vi "getType.vi"(8 "error in (no error)":errorcluster, 11 "Wire in":refnum<class "TextDecoration.lvclass">) -> (0 "error out":errorcluster, 2 "type":string, 3 "Wire out":refnum<class "TextDecoration.lvclass">)   [LabVIEW 2023, in "TLC_Scripto.lvlib" / "TextDecoration.lvclass"]
uses:
  TextDecoration.lvclass
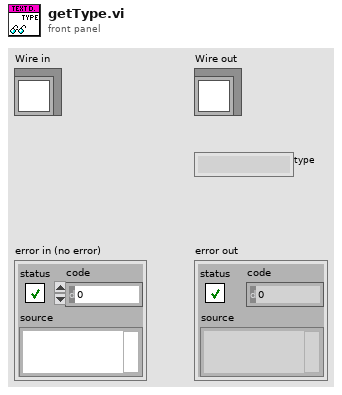
[diagram p1: front panel]
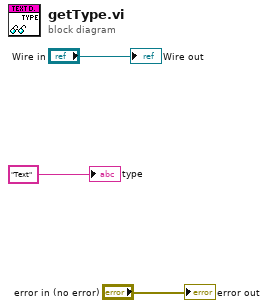
[diagram p0: block diagram]
diagram:
  "error out" <- "error in (no error)"
  "Wire out" <- "Wire in"
  "type" <- "Text"
